vi "mro apply Io Command (incomplete).vi"(8 "error in (no error)":errorcluster, 9 "status":i32, 10 "trig":i8, 11 "command":dbl) -> (0 "error out":errorcluster, 1 "status out":i32, 2 "function return":i8, 3 "command out":dbl)   [LabVIEW 2016]
doc: "MIRAOEXPORT MroBoolean MIRAOCALL mro_applyIoCommand( \n MroCommand command,\n MroBoolean trig,\n int* status\n );"
uses:
  mirao52e.dll
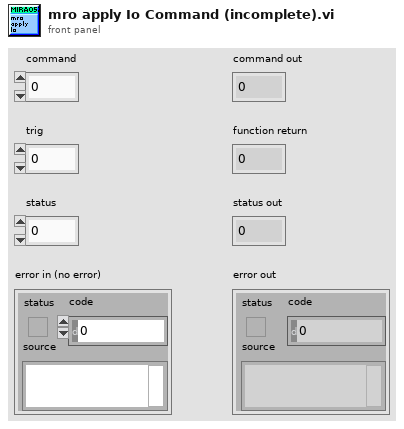
[diagram p1: front panel]
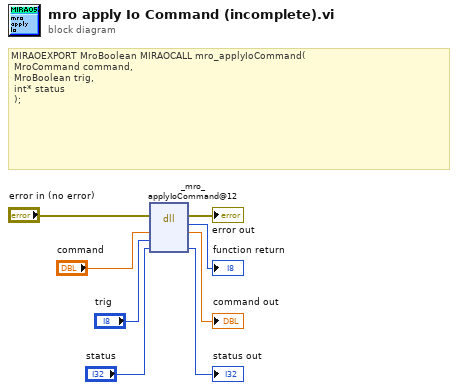
[diagram p0: block diagram]
diagram:
  # "MIRAOEXPORT MroBoolean MIRAOCALL mro_applyIoCommand( \n\tMroCommand command,\n\tMroBoolean trig,\n\tint* status\n\t);"
  n1 = dll-call lib="C:/Users/nvladim/Documents/Nikita-MDC/code/LabView/miraoDriver_32bit/mirao52e.*" fn="_mro_applyIoCommand@12"(error in="error in (no error)", "command"="command", "trig"="trig", "status"="status") -> (error out=→"error out":errorcluster, →"function return":i8, "command"=→"command out":dbl, "status"=→"status out":i32)  [unwired: 3 in, 1 out]
